vi "Add Renamed Files to Library.vi"(8 "error in":errorcluster, 10 "plugin library path":path, 11 "plugin files path":path[](array[path])) -> (0 "error out":errorcluster)   [LabVIEW 2021, in "InstrumentStudio Plug-In Editor.lvlib"]
uses:
  InstrumentStudio Plug-In Editor.lvlib
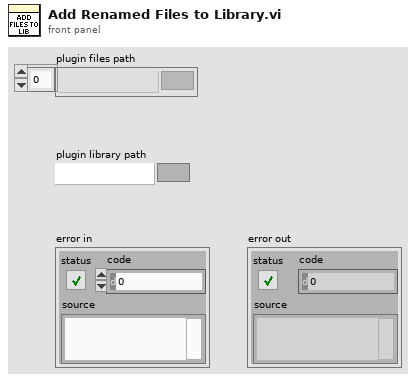
[diagram p1: front panel]
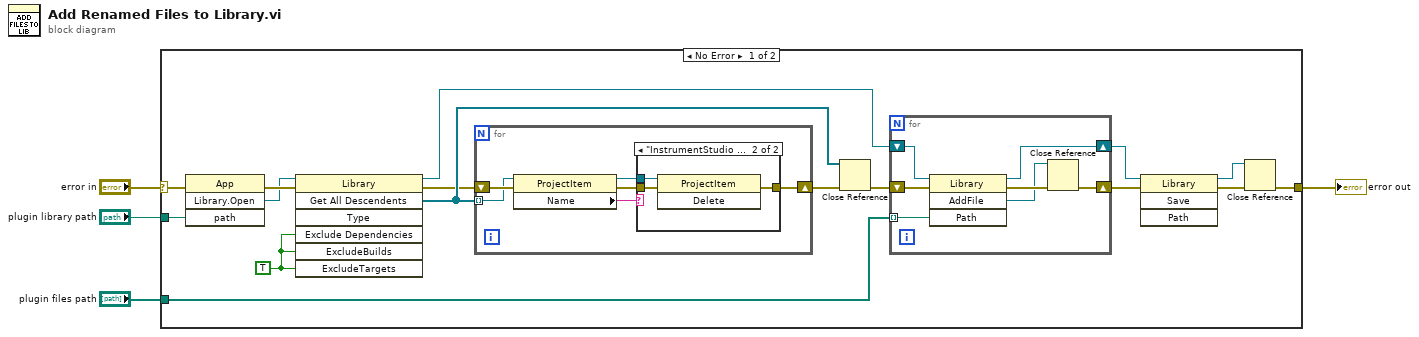
[diagram p0: block diagram]
diagram:
  n1 = case shown="No Error" "error in" {
    selector: "error in" -> [w20 w38]
    tunnel: "plugin library path" -> [w15 _]
    tunnel: "plugin files path" -> [w9 _]
    tunnel: [w5 w38] -> w1
    frame No Error {
      w12 = TRUE ("ExcludeDependencies")
      n2 = invoke class="App" method="Library.Open"(error in=w20, "path"=w15) -> (error out=w19:errorcluster, "Open Library"=w14:refnum<vi>)  [unwired: 2 in, 2 out]
      n3 = invoke class="Library" method="Get All Descendents"(reference=w14, error in=w19, "Exclude Dependencies"=w12, "ExcludeBuilds"=w12, "ExcludeTargets"=w12) -> (reference out=w10:refnum<vi>, error out=w16:errorcluster, "All Descendents"=w18:refnum<vi>[])  [unwired: 2 in, 4 out]
      n4 = for {
        shift-right: [w32] -> w17
        shift-left: w16 -> [w33]
        tunnel: w18 -> [w30] mode=indexing
        n5 = property class="ProjectItem"(reference=w30, error in=w33) -> (reference out=w29:refnum<vi>, error out=w31:errorcluster, "Name"=w28:string)
        n6 = case shown="\"InstrumentStudio Plug-In Template.gplugindata\", \"InstrumentStudio Plug-In Template.vi\"" w28 {
          tunnel: w31 -> [w34 w37]
          tunnel: [w34 w36] -> w32
          tunnel: w29 -> [_ w35]
          frame Default {
          }
          frame "InstrumentStudio Plug-In Template.gplugindata", "InstrumentStudio Plug-In Template.vi" {
            n7 = invoke class="ProjectItem" method="Delete"(reference=w35, error in=w37) -> (error out=w36:errorcluster)  [unwired: 1 in, 2 out]
          }
        }
      }
      n8 = Close Reference(reference=w18, error in (no error)=w17) -> (error out=w13:errorcluster)
      n9 = for {
        shift-right: [w25] -> w11
        shift-left: w13 -> [w27]
        shift-right: [w23] -> w7
        shift-left: w10 -> [w24]
        tunnel: w9 -> [w21] mode=indexing
        n10 = invoke class="Library" method="AddFile"(reference=w24, error in=w27, "Path"=w21) -> (reference out=w23:refnum<vi>, error out=w26:errorcluster, "AddFile"=w22:refnum<vi>)  [unwired: 1 in, 1 out]
        n11 = Close Reference(reference=w22, error in (no error)=w26) -> (error out=w25:errorcluster)
      }
      n12 = invoke class="Library" method="Save"(reference=w7, error in=w11) -> (reference out=w6:refnum<vi>, error out=w8:errorcluster)  [unwired: 2 in, 2 out]
      n13 = Close Reference(reference=w6, error in (no error)=w8) -> (error out=w5:errorcluster)
    }
    frame Error {
    }
  }
  "error out" <- w1
